vi "wait for 335(SubVI).vi"(8 "error in (no error)":errorcluster, 9 "Delay Time (s)":dbl=1.0, 10 "335 staus":refnum<queue>, 11 "abort":refnum<queue>) -> (0 "error out":errorcluster)   [LabVIEW 2019, in "SubVI.lvlib"]
uses:
  SubVI.lvlib
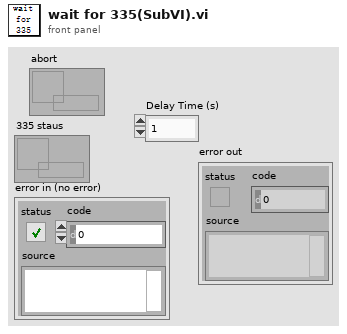
[diagram p1: front panel]
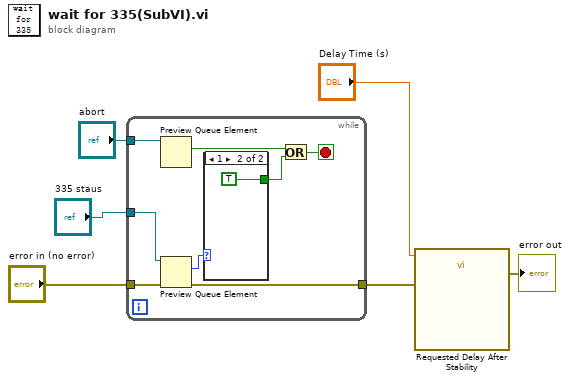
[diagram p0: block diagram]
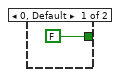
[diagram p2: hidden frame]
diagram:
  n1 = while {
    tunnel: "abort" -> [w14]
    tunnel: [w8] -> w5
    tunnel: "335 staus" -> [w11]
    tunnel: "error in (no error)" -> [w7]
    stop <- w12 stop-if-true
    n2 = Preview Queue Element(queue=w14) -> (element=w13:bool)  [unwired: 2 in, 3 out]
    n3 = Preview Queue Element(queue=w11, error in (no error)=w7) -> (element=w10:u16, error out=w8:errorcluster)  [unwired: 1 in, 2 out]
    n4 = case shown="1" w10 {
      tunnel: [FALSE TRUE] -> w9
      frame 0, Default {
      }
      frame 1 {
      }
    }
    n5 = Or(x=w13, y=w9) -> (x .or. y?=w12:bool)
  }
  n6 = call "Requested Delay After Stability"("error in (no error)"=w5, "Delay Time (s)"="Delay Time (s)") -> ("error out"=→"error out":errorcluster)  [unwired: 9 in]
